vi "Read I2C Slave Address (0x40).vi"(8 "error in (no error)":errorcluster, 11 "LINX-PCA9865 PWM in":refnum<class "LINX-PCA9685 PWM.lvclass">) -> (0 "error out":errorcluster, 2 "I2C Slave Address (0x40)":u8=64 format="%.0x", 3 "LINX-PCA9865 PWM out":refnum<class "LINX-PCA9685 PWM.lvclass">)   [LabVIEW 2020, in "LINX-PCA9685 PWM.lvclass"]
uses:
  LINX-PCA9685 PWM.lvclass
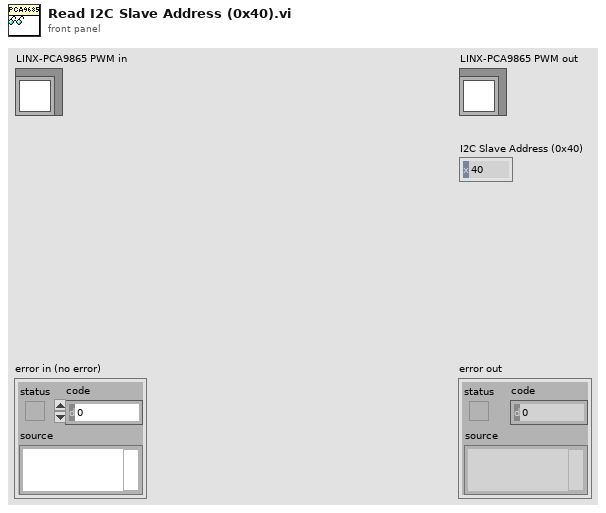
[diagram p1: front panel]
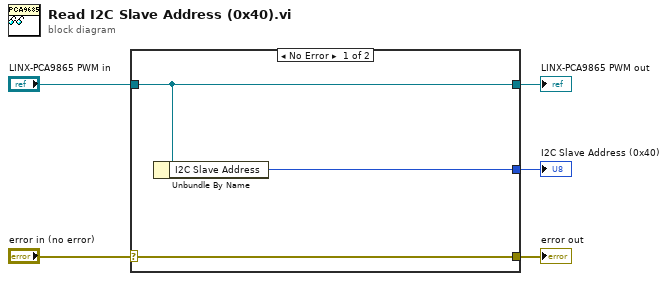
[diagram p0: block diagram]
diagram:
  n1 = case shown="No Error" "error in (no error)" {
    selector: "error in (no error)" -> [w8 w9]
    tunnel: [w8 w9] -> w4
    tunnel: [w7 w10] -> w2
    tunnel: "LINX-PCA9865 PWM in" -> [w7 w10]
    tunnel: [w6 _] -> w1
    frame No Error {
      n2 = Unbundle By Name(w7) -> ("I2C Slave Address"=w6:u8)
    }
    frame Error {
    }
  }
  "error out" <- w4
  "LINX-PCA9865 PWM out" <- w2
  "I2C Slave Address (0x40)" <- w1
